vi "E8257C_local.vi"(1 "error in":errorcluster, 2 "GPIB address":string="19") -> (0 "error out":errorcluster)   [LabVIEW 2011]
panel:
  # "This VI controls Agilent E8257C PSG Analog Signal Generator \n  Set to LOCAL state"
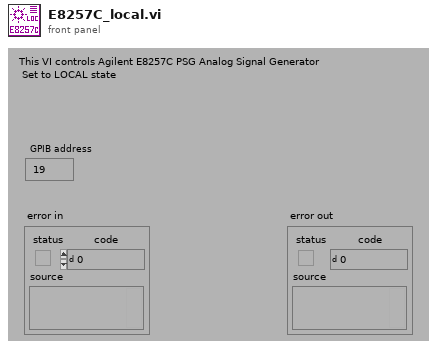
[diagram p1: front panel]
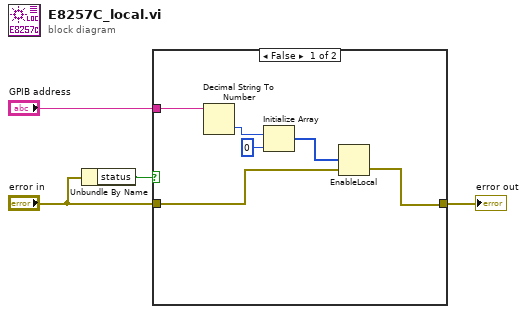
[diagram p0: block diagram]
diagram:
  n1 = Unbundle By Name("error in") -> ("status"=w4:bool)
  n2 = case shown="False" w4 {
    tunnel: "error in" -> [w10 w11]
    tunnel: [w9 w11] -> w2
    tunnel: "GPIB address" -> [w8 _]
    frame False {
      n3 = Decimal String To Number(string=w8) -> (number=w7:i32)  [unwired: 2 in, 1 out]
      n4 = Initialize Array(w7, 0 ("dimension size")) -> (w5:i32[])
      n5 = EnableLocal(2:w10, 3:w5) -> (0:w9:errorcluster)  [unwired: 1 in, 1 out]
    }
    frame True {
    }
  }
  "error out" <- w2
